vi "read TBM configuration.vi"(8 "error in":errorcluster, 11 "Watchdog editor node in":refnum<class "Watchdog editor node.lvclass">) -> (0 "error out":errorcluster, 2 "configuration":refnum<class "TBM configuration.lvclass">, 3 "Watchdog editor node out":refnum<class "Watchdog editor node.lvclass">)   [LabVIEW 2013, in "Watchdog editor node.lvclass"]
uses:
  Watchdog editor node.lvclass
  <vilib>/NI/Tag Bus Module Framework/root configuration/TBM configuration.lvclass
  Watchdog editor node.lvclass/Watchdog editor node.ctl
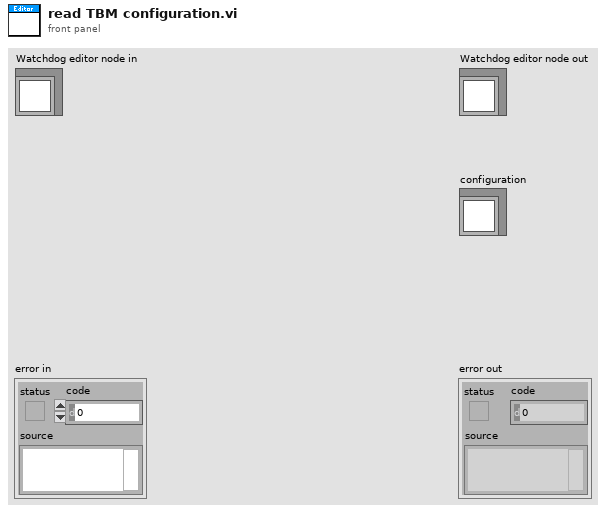
[diagram p1: front panel]
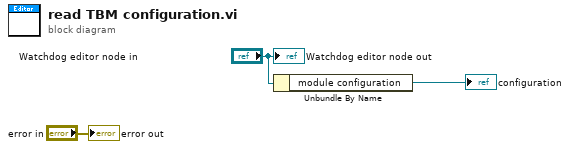
[diagram p0: block diagram]
diagram:
  n1 = Unbundle By Name("Watchdog editor node in") -> ("module configuration"=→"configuration":refnum<class "Watchdog configuration.lvclass">)
  "error out" <- "error in"
  "Watchdog editor node out" <- "Watchdog editor node in"
